vi "Actor Core.vi"(8 "error in (no error)":errorcluster, 11 "Operator UI.lvclass":refnum<class "Measurement UI.lvclass">) -> (0 "error out":errorcluster, 3 "Actor Framework.lvlib:Actor":refnum<class "Actor.lvclass">)   [LabVIEW 2015, in "Measurement UI.lvlib" / "Measurement UI.lvclass"]
doc: "This is Actor Core.vi, the main message handling loop for Actors. An actor usually just sits in this loop and processes messages as they arrive. Any error returned by the message Do.vi call will stop the loop, with error code 43 as the cannonical signal to stop with no error sent to caller. Descendants may override that in Handle Error.vi."
uses:
  Measurement UI.lvclass
  <vilib>/ActorFramework/Actor/Actor.lvclass
  <vilib>/ActorFramework/Actor/Actor.lvclass/Actor.ctl
  <vilib>/ActorFramework/Message Enqueuer/Message Enqueuer.lvclass/Message Enqueuer.ctl
  <vilib>/ActorFramework/Message Enqueuer/Init from Existing Queue.vi
  <vilib>/ActorFramework/Message Enqueuer/Enqueue.vi
  Accessors/Write Digitizer.vi
  Accessors/Write Function Generator.vi
  Accessors/Write Load New Measurement.vi
  Accessors/Write Measurement.vi
  Accessors/Write Multimeter.vi
  Accessors/Write Power Supply.vi
  Accessors/Write Results Listbox.vi
  Accessors/Write Run.vi
  Accessors/Write Show FP_.vi
  Accessors/Write Status Display.vi
  Accessors/Write Stop Button.vi
  Accessors/Write Tab Control.vi
  Accessors/Write View Results.vi
  <vilib>/ActorFramework/Message Priority Queue/Priority Enqueue.vi
  <vilib>/ActorFramework/Message Enqueuer/Message Enqueuer.lvclass
  <vilib>/ActorFramework/Stop Msg/Stop Msg.lvclass
  Messages/Ask Controller to Launch Results UI Msg/Ask Controller to Launch Results UI Msg.lvclass
  User Interface/UI.lvclass
  Messages/Send Run Measurement Message/Send Run Measurement Message.lvclass
  Messages/Send Get Hardware Info Message/Send Get Hardware Info Message.lvclass
  Messages/Check Run Button/Check Validity of Selection.lvclass
  Messages/Prompt User for Path to load/Prompt User for File Path to Load From.lvclass
panel:
  in  "about":bool
  in  "Load New Measurement":bool
  in  "Show FP?":bool
  in  "Stop Button":bool
  in  "Run":bool
  in  "Power Supply":u16(ring)
  in  "Function Generator":u16(ring)
  in  "Digitizer":u16(ring)
  in  "Multimeter":u16(ring)
  in  "Tab Control":enum32{"Test Status", "Results"}(tab)
  in  "Status Display":string
  in  "View Results":bool
  in  "Results Listbox":i32(listbox)
  in  "Measurement":u16(ring)
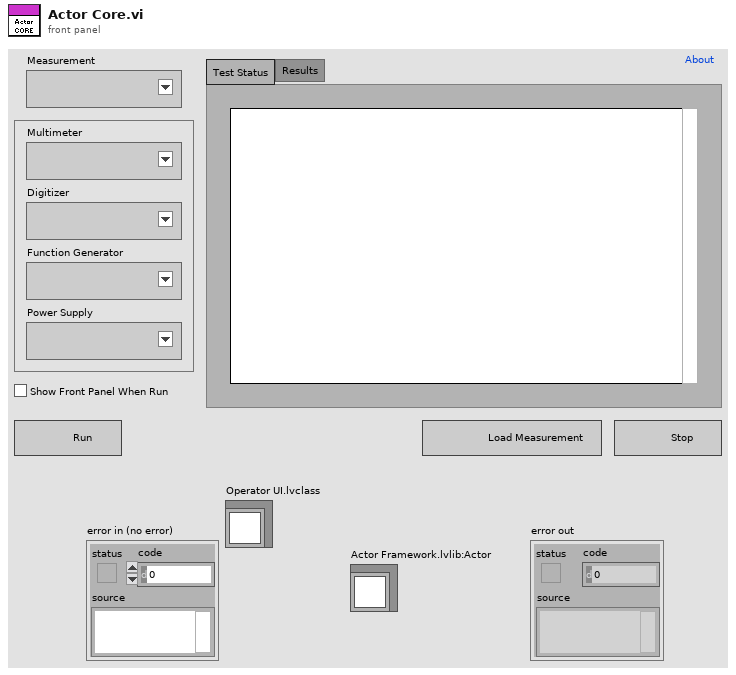
[diagram p1: front panel]
types:
  T1 = enum8{"Enabled", "Disabled", "Disabled and Grayed Out"}
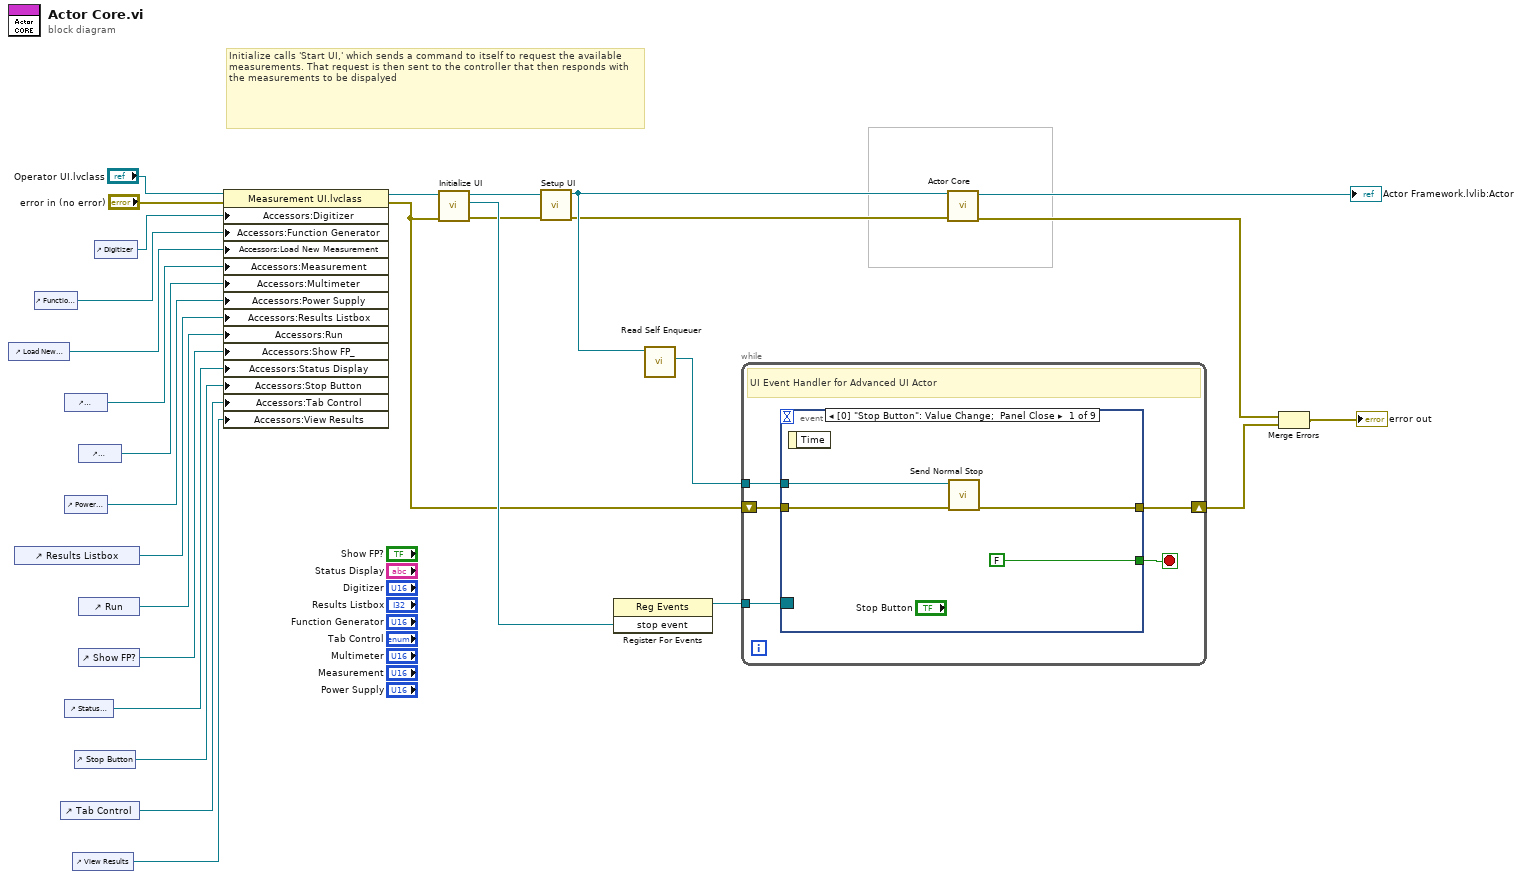
[diagram p0: block diagram]
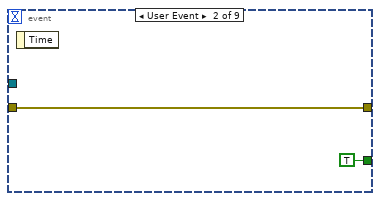
[diagram p2: hidden frame]
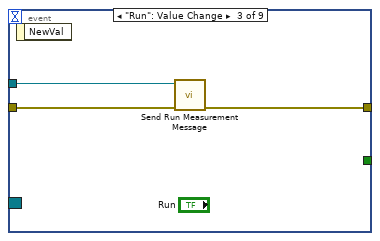
[diagram p3: hidden frame]
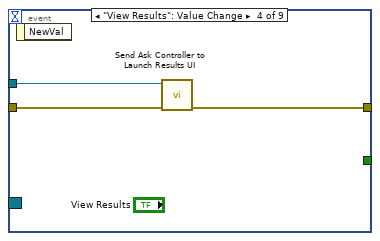
[diagram p4: hidden frame]
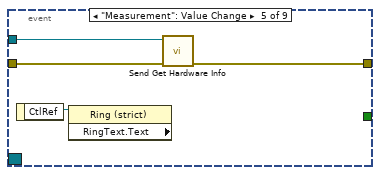
[diagram p5: hidden frame]
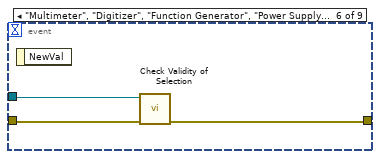
[diagram p6: hidden frame]
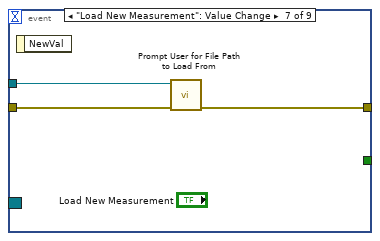
[diagram p7: hidden frame]
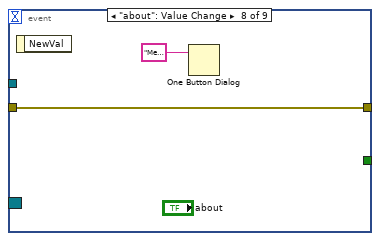
[diagram p8: hidden frame]
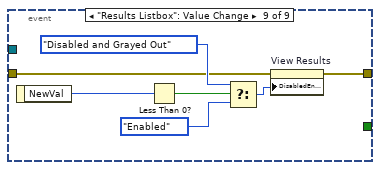
[diagram p9: hidden frame]
diagram:
  # "Initialize calls 'Start UI,' which sends a command to itself to request the available measurements. That request is then sent to the controller that then responds with the measurements to be dispalyed"
  n1 = control-ref of="Load New Measurement"() -> (w11:refnum<vi>)
  n2 = control-ref of="Results Listbox"() -> (w15:refnum<vi>)
  n3 = control-ref of="Function Generator"() -> (w12:refnum<vi>)
  n4 = control-ref of="Tab Control"() -> (w17:refnum<vi>)
  n5 = control-ref of="Measurement"() -> (w10:refnum<vi>)
  n6 = control-ref of="Power Supply"() -> (w14:refnum<vi>)
  n7 = control-ref of="Status Display"() -> (w19:refnum<vi>)
  n8 = control-ref of="View Results"() -> (w16:refnum<vi>)
  n9 = control-ref of="Stop Button"() -> (w18:refnum<vi>)
  n10 = control-ref of="Multimeter"() -> (w9:refnum<vi>)
  n11 = control-ref of="Run"() -> (w8:refnum<vi>)
  n12 = control-ref of="Show FP?"() -> (w20:refnum<vi>)
  n13 = control-ref of="Digitizer"() -> (w13:refnum<vi>)
  n14 = property class="Measurement UI.lvclass"(reference="Operator UI.lvclass", error in="error in (no error)", "Accessors:Digitizer"=w13, "Accessors:Function Generator"=w12, "Accessors:Load New Measurement"=w11, "Accessors:Measurement"=w10, "Accessors:Multimeter"=w9, "Accessors:Power Supply"=w14, "Accessors:Results Listbox"=w15, "Accessors:Run"=w8, "Accessors:Show FP_"=w20, "Accessors:Status Display"=w19, "Accessors:Stop Button"=w18, "Accessors:Tab Control"=w17, "Accessors:View Results"=w16) -> (reference out=w6:refnum<class "Measurement UI.lvclass">, error out=w3:errorcluster)
  n15 = call "Initialize UI.vi"("error in (no error)"=w3, "UI in"=w6) -> ("error out"=w4:errorcluster, "stop event"=w22:refnum<user-event>, "UI out"=w5:refnum<class "Measurement UI.lvclass">)  [unwired: 7 in]
  n16 = call-dynamic "Setup UI.vi"("error in (no error)"=w4, "Operator UI in"=w5) -> ("error out"=w1:errorcluster, "Operator UI out"=w2:refnum<class "Measurement UI.lvclass">)  [unwired: 8 in]
  n17 = register-events(w22) -> (reference out=w23:refnum<event-registration>)  [unwired: 2 in, 1 out]
  n18 = call <vilib>:"Read Self Enqueuer.vi"("Actor"=w2) -> ("Self Enqueuer"=w27:refnum<class "Message Enqueuer.lvclass">)  [unwired: 10 in]
  n19 = while {
    tunnel: w27 -> [w32]
    tunnel: w23 -> [w31]
    shift-right: [w29] -> w26
    shift-left: w3 -> [w30]
    stop <- w33 stop-if-true
    # "UI Event Handler for Advanced UI Actor"
    n20 = event shown="[0] \"Stop Button\": Value Change;  Panel Close" {
      selector: w31 -> [_ _ _ _ _ _ _ _ _]
      dyn-events: _ -> [_ _ _ _ _ _ _ _ _]
      timeout: _ -> [_ _ _ _ _ _ _ _ _]
      tunnel: [FALSE TRUE _ _ _ _ _ _ _] -> w33
      tunnel: w32 -> [w36 _ w42 w45 w49 w52 w55 _ _]
      tunnel: w30 -> [w35 w38 w41 w44 w48 w51 w54 w56 w59]
      tunnel: [w34 w38 w40 w43 w47 w50 w53 w56 w58] -> w29
      event "Stop Button": Value Change; Panel Close {
        n21 = event-data() -> ()  [unwired: 1 in, 1 out]
        n22 = call <vilib>:"Send Normal Stop.vi"("error in (no error)"=w35, "Message Enqueuer"=w36) -> ("error out"=w34:errorcluster)  [unwired: 9 in]
      }
      event User Event {
        n23 = event-data() -> ()  [unwired: 1 in, 1 out]
      }
      event "Run": Value Change {
        n24 = event-data() -> ()  [unwired: 1 in, 1 out]
        n25 = call "Send Run Measurement Message.vi"("error in (no error)"=w41, "Message Enqueuer in"=w42) -> ("error out"=w40:errorcluster)  [unwired: 8 in, 1 out]
      }
      event "View Results": Value Change {
        n26 = event-data() -> ()  [unwired: 1 in, 1 out]
        n27 = call "Send Ask Controller to Launch Results UI.vi"("error in (no error)"=w44, "Message Enqueuer in"=w45) -> ("error out"=w43:errorcluster)  [unwired: 8 in, 1 out]
      }
      event "Measurement": Value Change {
        n28 = event-data() -> ("CtlRef"=w46:refnum<vi>)  [unwired: 1 in]
        n29 = property class="Ring (strict)" props=["RingText", "Text"](reference=w46) -> ()  [unwired: 1 in, 3 out]
        n30 = call "Send Get Hardware Info.vi"("error in (no error)"=w48, "Message Enqueuer in"=w49) -> ("error out"=w47:errorcluster)  [unwired: 8 in, 1 out]
      }
      event "Multimeter", "Digitizer", "Function Generator", "Power Supply": Value Change {
        n31 = event-data() -> ()  [unwired: 1 in, 1 out]
        n32 = call "Check Validity of Selection.vi"("error in (no error)"=w51, "Message Enqueuer in"=w52) -> ("error out"=w50:errorcluster)  [unwired: 8 in, 1 out]
      }
      event "Load New Measurement": Value Change {
        n33 = event-data() -> ()  [unwired: 1 in, 1 out]
        n34 = call "Prompt User for File Path to Load From.vi"("error in (no error)"=w54, "Message Enqueuer in"=w55) -> ("error out"=w53:errorcluster)  [unwired: 8 in, 1 out]
      }
      event "about": Value Change {
        n35 = event-data() -> ()  [unwired: 1 in, 1 out]
        n36 = One Button Dialog(message="Measurement Manager v2.0\n\nNational Instruments (C) 2013\nWritten in NI LabVIEW 2012 by Elijah Kerry \nElijah.Kerry@ni.com\n\nni.com/largeapps\nekerry.wordpress.com") -> ()  [unwired: 1 in, 1 out]
      }
      event "Results Listbox": Value Change {
        n37 = event-data() -> ("NewVal"=w60:i32)  [unwired: 1 in]
        n38 = Less Than 0?(x=w60) -> (x < 0?=w61:bool)
        n39 = Select(t=T1."Disabled and Grayed Out" ("Disabled"), s=w61, f=T1."Enabled" ("Disabled")) -> (s? t:f=w64:T1)
        n40 = property on="View Results" class="Bool"(error in=w59, "DisabledEnum"=w64) -> (error out=w58:errorcluster)  [unwired: 1 in, 1 out]
      }
    }
  }
  n41 = call-parent "Actor Core.vi"("error in"=w1, "User Interface"=w2) -> ("error out"=w25:errorcluster, "Actor out"=→"Actor Framework.lvlib:Actor":refnum<class "Actor.lvclass">)  [unwired: 8 in]
  n42 = Merge Errors(w25, w26) -> (→"error out":errorcluster)
